vi "LoggingBlock Backup to be deleted later.vi"(8 "error in":errorcluster, 9 "Data In":T2, 11 "Queue Ref":T1) -> (0 "error out":errorcluster)   [LabVIEW 2014]
uses:
  TypeDef/Q1 Message.ctl
  <vilib>/Platform/TimedLoop/XDataNode/timing_clust.ctl
  <vilib>/Platform/TimedLoop/XDataNode/nitl_modes.ctl
  <vilib>/Platform/TimedLoop/XDataNode/wakeup.ctl
  <vilib>/platform/TimedLoop/XDataNode/XDataNode.xnode
  <vilib>/Platform/TimedLoop/XDataNode/XDNodeRunTimeDep.lvlib
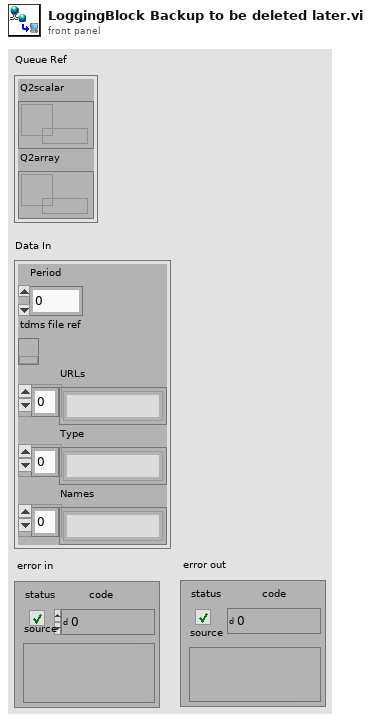
[diagram p1: front panel]
types:
  T1 = cluster{"Q2scalar":refnum<queue>, "Q2array":refnum<queue>}
  T2 = cluster{"Period":i64, "tdms file ref":refnum<k34>, "URLs":string[], "Type":string[], "Names":string[]}
  T3 = typedef "Q1 Message.ctl" = cluster{"state":enum16{"initialize 1", "initialize 2", "initialize 3", "initialize 4", "idle", "preparation", "record", "stop", "exit", "defrag", "View", "Create Database"}, "data":variant}
  T4 = typedef "XDNodeRunTimeDep.lvlib/timing_clust.ctl" = cluster{"Expected End [f-1]":u64, "Actual End [f-1]":u64, "Finished Late? [f-1]":bool, "Expected End [i-1]":u64, "Actual End [i-1]":u64, "Finished Late? [i-1]":bool, "Expected Start [i]":u64, "Actual Start [i]":u64, "Expected Start [f]":u64, "Actual Start [f]":u64, "Source Name":string, "Structure Name":string, "Period":i64, "Deadline":i64, "Offset":i64, "Start":i64, "Priority":i32, "Timeout":i32, "Mode":T5, "Wakeup Reason":T6, "Error":errorcluster, "Source Type":string, "Secondary Source Type":string, "Global End Time":u64, "Global Start Time":u64, "Frame Duration":u64, "Iteration Duration":u64, "Assigned CPU":i32, "I/O Scan Engine Mode":u32}
  T5 = typedef "XDNodeRunTimeDep.lvlib/nitl_modes.ctl" = enum32{"No Change", "Process missed periods, maintain original phase", "Discard missed periods, maintain original phase", "Process missed periods, ignore original phase", "Discard missed periods, ignore original phase"}
  T6 = typedef "XDNodeRunTimeDep.lvlib/wakeup.ctl" = enum32{"Normal", "Aborted", "Asynchronous wakeup", "Timing source error", "Timed loop error", "Timeout"}
  T7 = enum16{"initialize 1", "initialize 2", "initialize 3", "initialize 4", "idle", "preparation", "record", "stop", "exit", "defrag", "View", "Create Database"}
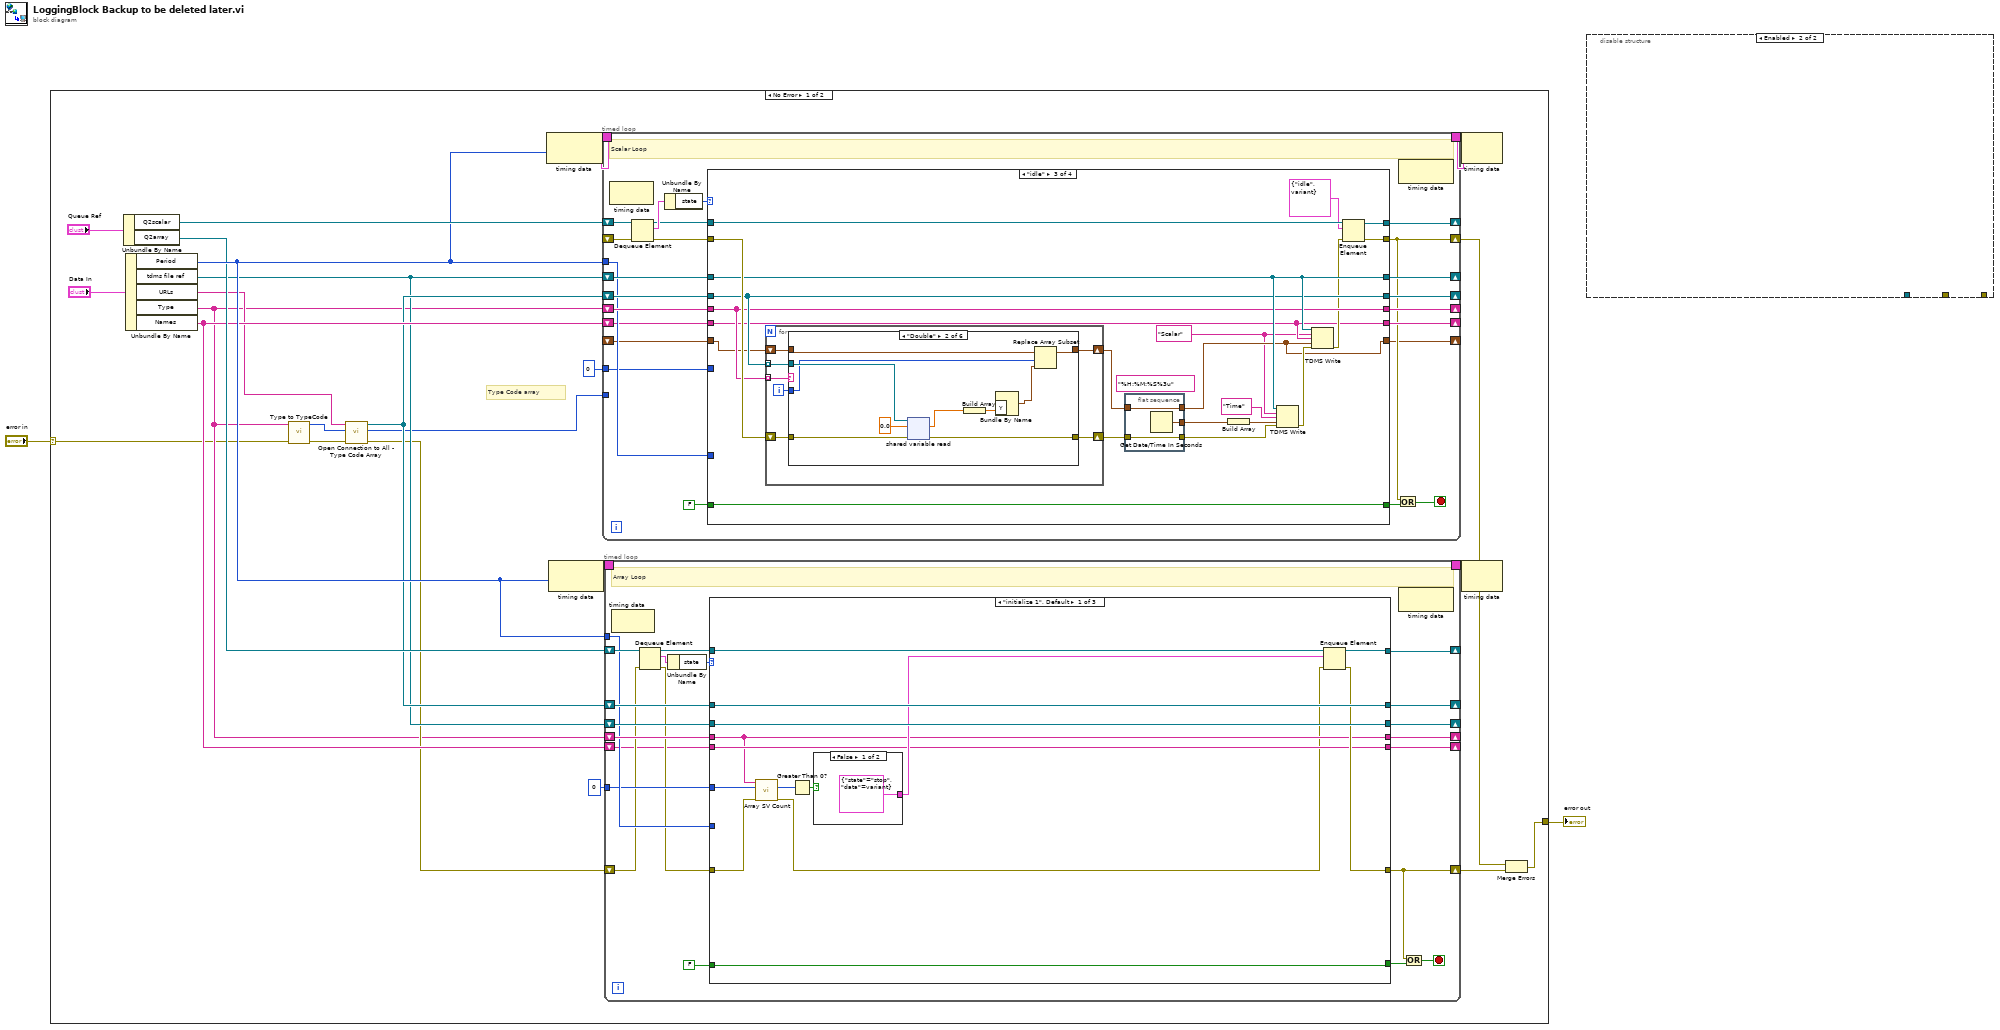
[diagram p0: block diagram]
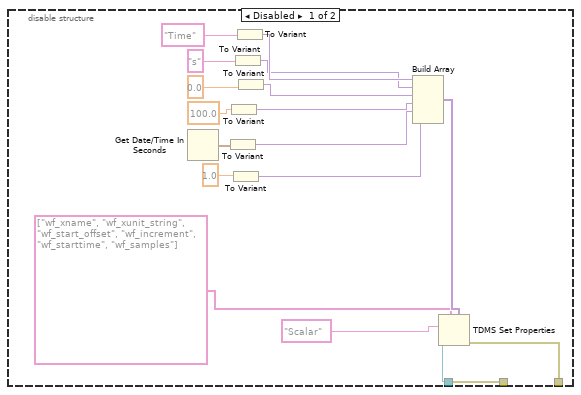
[diagram p2: hidden frame]
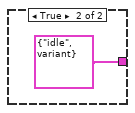
[diagram p3: hidden frame]
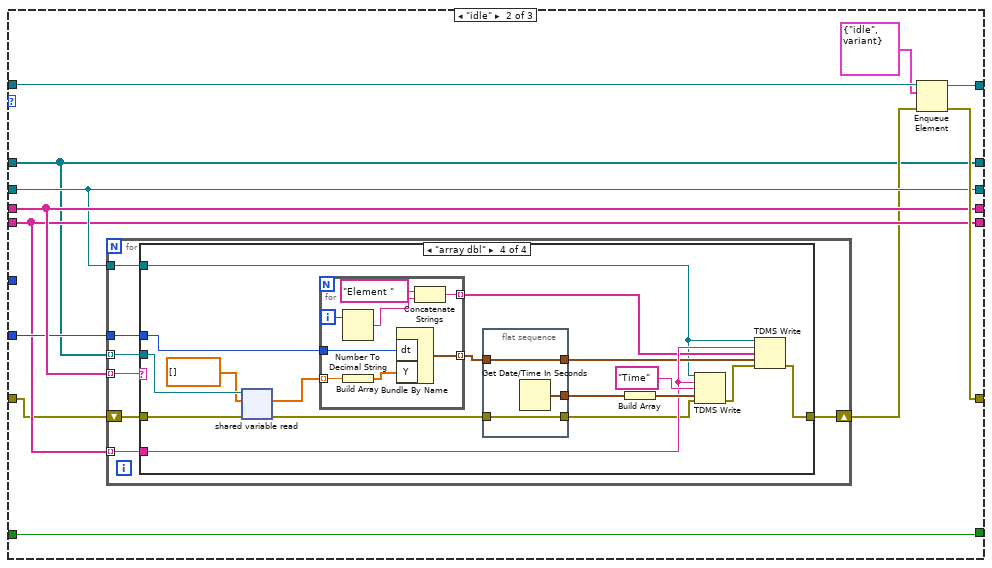
[diagram p4: hidden frame]
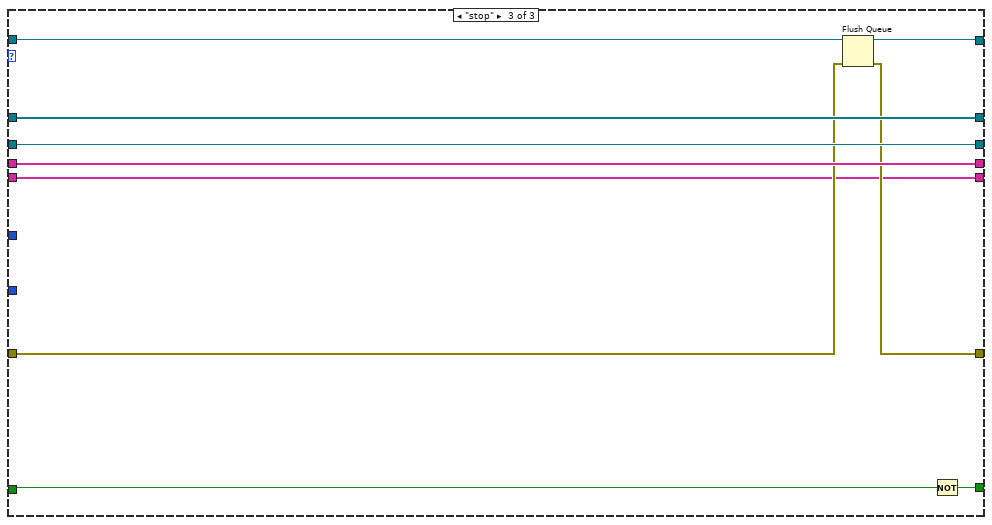
[diagram p8: hidden frame]
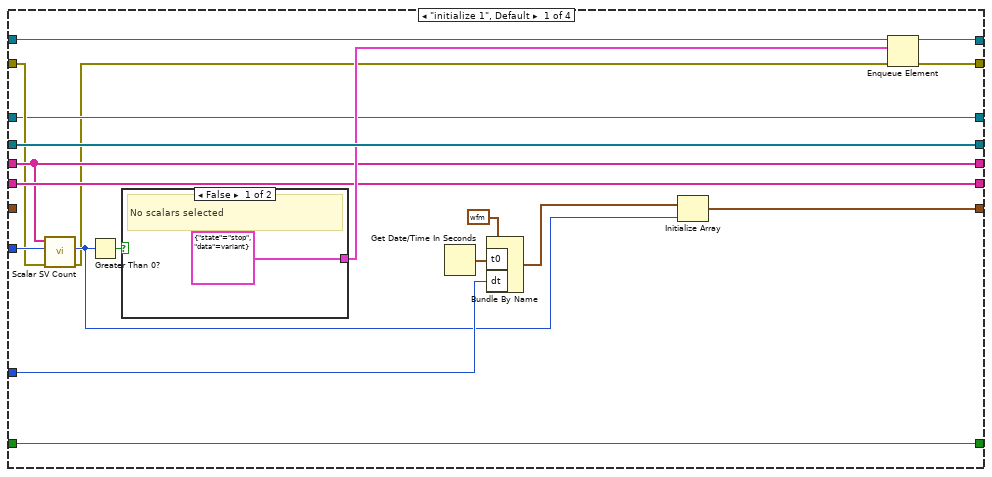
[diagram p9: hidden frame]
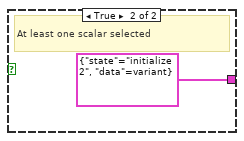
[diagram p10: hidden frame]
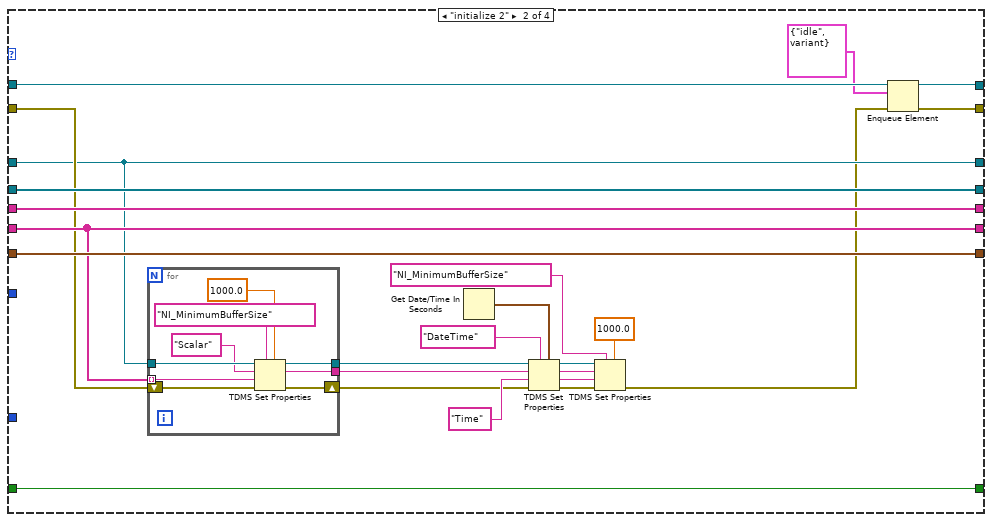
[diagram p11: hidden frame]
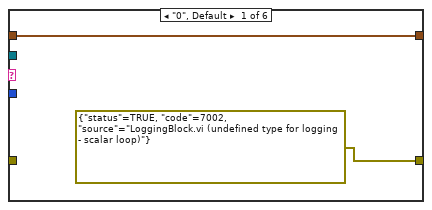
[diagram p12: hidden frame]
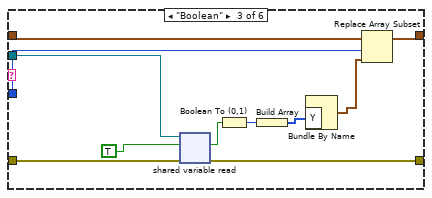
[diagram p13: hidden frame]
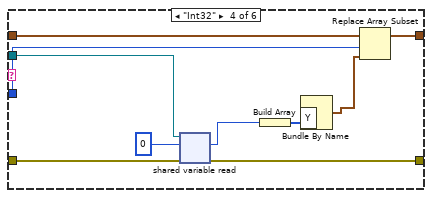
[diagram p14: hidden frame]
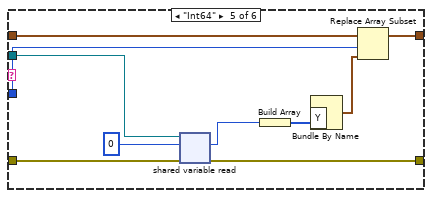
[diagram p15: hidden frame]
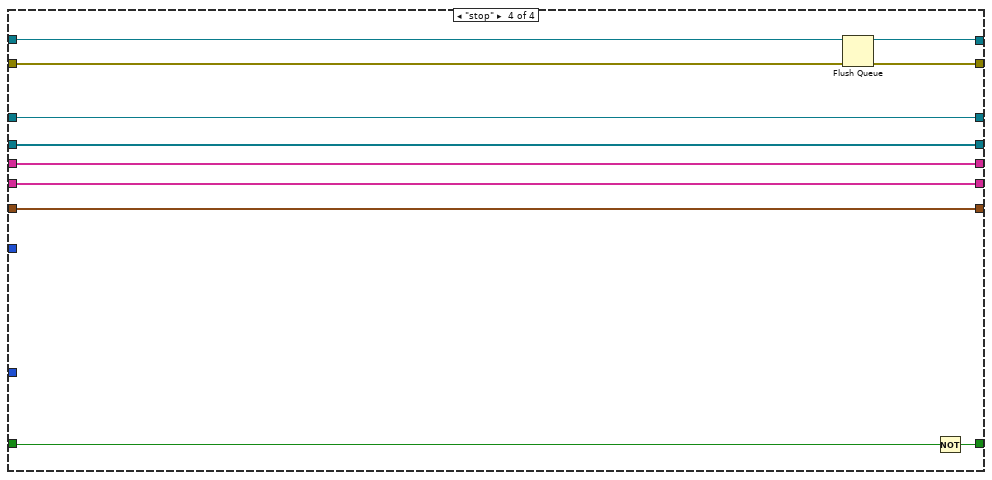
[diagram p17: hidden frame]
diagram:
  n1 = case shown="No Error" "error in" {
    selector: "error in" -> [w6 w300]
    tunnel: [w13 w300] -> w1
    frame No Error {
      # "Type Code array"
      n2 = Unbundle By Name("Queue Ref") -> ("Q2scalar"=w22:refnum<queue>, "Q2array"=w17:refnum<queue>)
      n3 = Unbundle By Name("Data In") -> ("Period"=w18:i64, "tdms file ref"=w9:refnum<k34>, "URLs"=w11:string[], "Type"=w7:string[], "Names"=w12:string[])
      n4 = call "Type to TypeCode.vi"("Error In"=w6, "Type Array"=w7) -> ("Error Out"=w5:errorcluster, "Type code Array"=w4:i32[])  [unwired: 7 in, 1 out]
      n5 = call "Open Connection to All - Type Code Array.vi"("Error In"=w5, "Type code Array"=w4, "URL array"=w11) -> ("Error Out"=w8:errorcluster, "Type code Array dup"=w3:i32[], "Array of SV Refnums"=w10:refnum<k21>[])  [unwired: 5 in, 1 out]
      n6 = node-c288(w18) -> (w24:T4)
      n7 = node-c288(w18) -> (w20:T4)
      n8 = timed-loop {
        timing: w24 -> [_]
        timing-out: [_] -> w23
        shift-right: [w143] -> _
        shift-left: w10 -> [w146]
        shift-right: [w141] -> _
        shift-left: w7 -> [w152]
        shift-right: [w144] -> _
        shift-left: w9 -> [w145]
        shift-right: [w133] -> w15
        shift-left: _ -> [w139]
        tunnel: w18 -> [w142]
        shift-right: [w147] -> _
        shift-left: w22 -> [w150]
        tunnel: 0 -> [w140]
        shift-right: [w136] -> _
        shift-left: w12 -> [w137]
        shift-right: [w131] -> _
        shift-left: _ -> [w130]
        tunnel: w3 -> [_]
        stop <- w132 stop-if-true
        # "Scalar Loop"
        n9 = node-c288() -> ()  [unwired: 1 in, 1 out]
        n10 = Dequeue Element(queue=w150, error in (no error)=w139) -> (queue out=w148:refnum<queue>, element=w151:T3, error out=w138:errorcluster)  [unwired: 1 in, 1 out]
        n11 = Unbundle By Name(w151) -> ("state"=w149:T7)
        n12 = case shown="\"idle\"" w149 {
          tunnel: w138 -> [w161 w185 w227 w289]
          tunnel: w146 -> [w169 w195 w217 w292]
          tunnel: w152 -> [w162 w192 w216 w291]
          tunnel: [w166 w194 w214 w288] -> w133
          tunnel: w148 -> [w171 w197 w221 w290]
          tunnel: [w170 w196 w220 w287] -> w147
          tunnel: [w164 w193 w210 w285] -> w134
          tunnel: [w155 w184 w218 w293] -> w144
          tunnel: w145 -> [w155 w184 w218 w293]
          tunnel: [w169 w195 w217 w292] -> w143
          tunnel: w142 -> [w157 _ _ _]
          tunnel: [w162 w192 w216 w291] -> w141
          tunnel: w140 -> [w163 _ _ _]
          tunnel: w137 -> [w165 w186 w213 w286]
          tunnel: [w165 w186 w213 w286] -> w136
          tunnel: FALSE -> [w164 w193 w210 w284]
          tunnel: [w160 w187 w208 w283] -> w131
          tunnel: w130 -> [_ w187 w209 w283]
          frame "initialize 1", Default {
            n13 = call "Scalar SV Count.vi"("Error In"=w161, "Initial number"=w163, "Type array"=w162) -> ("Error Out"=w153:errorcluster, "Number of scalar SV"=w154:i32)  [unwired: 7 in]
            n14 = Greater Than 0?(x=w154) -> (x > 0?=w168:bool)
            n15 = case shown="False" w168 {
              tunnel: [T3 {"state"=enum."stop", "data"=variant} ("Q1 Message") T3 {"state"=enum."initialize 2", "data"=variant} ("Q1 Message")] -> w167
              frame False {
                # "No scalars selected"
              }
              frame True {
                # "At least one scalar selected"
              }
            }
            n16 = Get Date/Time In Seconds() -> (seconds since 1Jan1904=w158:timestamp)
            n17 = Bundle By Name(cluster=waveform(dbl) {"t0"=timestamp(0 s since 1904-01-01), "dt"=1.0, "Y"=[]}, "t0"=w158, "dt"=w157) -> (w156:waveform(dbl))
            n18 = Initialize Array(w156, w154) -> (w160:waveform(dbl)[])
            n19 = Enqueue Element(queue=w171, element=w167, error in (no error)=w153) -> (queue out=w170:refnum<queue>, error out=w166:errorcluster)  [unwired: 1 in, 1 out]
          }
          frame "initialize 2" {
            n20 = for {
              tunnel: w186 -> [w206] mode=indexing
              tunnel: w184 -> [w204]
              shift-right: [w200] -> w182
              shift-left: w185 -> [w205]
              tunnel: [w199] -> w183
              tunnel: [w198] -> w180
              n21 = TDMS Set Properties(5:1000.0, 7:"NI_MinimumBufferSize", 8:w205, 9:w206, 10:"Scalar", 11:w204) -> (0:w200:errorcluster, 2:w199:string, 3:w198:refnum<k34>)  [unwired: 1 out]
            }
            n22 = Get Date/Time In Seconds() -> (seconds since 1Jan1904=w190:timestamp)
            n23 = TDMS Set Properties(5:w190, 7:"DateTime" ("property names"), 8:w182, 9:"Time", 10:w183, 11:w180) -> (0:w177:errorcluster, 1:w178:string, 2:w179:string, 3:w181:refnum<k34>)
            n24 = TDMS Set Properties(5:1000.0, 7:"NI_MinimumBufferSize", 8:w177, 9:w178, 10:w179, 11:w181) -> (0:w174:errorcluster)  [unwired: 3 out]
            n25 = Enqueue Element(queue=w197, element=T3 {"state"=enum."idle", "data"=variant} ("Q1 Message"), error in (no error)=w174) -> (queue out=w196:refnum<queue>, error out=w194:errorcluster)  [unwired: 1 in, 1 out]
          }
          frame "idle" {
            (unwired) "%H:%M:%S%3u" ("time format string (%c)")
            w207 = "Scalar"
            n26 = for {
              tunnel: w217 -> [w237] mode=indexing
              tunnel: w216 -> [w232] mode=indexing
              shift-right: [w235] -> w226
              shift-left: w227 -> [w236]
              shift-right: [w233] -> w225
              shift-left: w209 -> [w234]
              i -> [w231]
              n27 = case shown="\"Double\"" w232 {
                tunnel: w237 -> [_ w244 w258 w263 w275 _]
                tunnel: w236 -> [_ w246 w260 w267 w277 w281]
                tunnel: [errorcluster {"status"=TRUE, "code"=7002, "source"="LoggingBlock.vi (undefined type for logging - scalar loop)"} ("error out") w245 w259 w266 w276 w281] -> w235
                tunnel: w234 -> [w239 w242 w256 w264 w272 w282]
                tunnel: [w239 w243 w257 w265 w271 w282] -> w233
                tunnel: w231 -> [_ w241 w255 w261 w273 _]
                frame "0", Default {
                }
                frame "Double" {
                  n28 = shared-variable-read(w244, w246, 0.0) -> (w245:errorcluster, w247:dbl)  [unwired: 2 out]
                  n29 = Build Array(w247) -> (w248:dbl[])
                  n30 = Bundle By Name("Y"=w248) -> (w240:waveform(dbl))  [unwired: 1 in]
                  n31 = Replace Array Subset(array=w242, new element=w240, index=w241) -> (w243:waveform(dbl)[])
                }
                frame "Boolean" {
                  n32 = shared-variable-read(w258, w260, TRUE) -> (w259:errorcluster, w251:bool)  [unwired: 2 out]
                  n33 = Boolean To (0,1)(Boolean=w251) -> (0, 1=w252:i16)
                  n34 = Build Array(w252) -> (w250:i16[])
                  n35 = Bundle By Name("Y"=w250) -> (w254:waveform(i16))  [unwired: 1 in]
                  n36 = Replace Array Subset(array=w256, new element=w254, index=w255) -> (w257:waveform(dbl)[])
                }
                frame "Int32" {
                  n37 = shared-variable-read(w263, w267, 0) -> (w266:errorcluster, w268:i32)  [unwired: 2 out]
                  n38 = Build Array(w268) -> (w269:i32[])
                  n39 = Bundle By Name("Y"=w269) -> (w262:waveform(i32))  [unwired: 1 in]
                  n40 = Replace Array Subset(array=w264, new element=w262, index=w261) -> (w265:waveform(dbl)[])
                }
                frame "Int64" {
                  n41 = shared-variable-read(w275, w277, i64 0) -> (w276:errorcluster, w278:i64)  [unwired: 2 out]
                  n42 = Build Array(w278) -> (w279:i64[])
                  n43 = Bundle By Name("Y"=w279) -> (w274:waveform(i64))  [unwired: 1 in]
                  n44 = Replace Array Subset(array=w272, new element=w274, index=w273) -> (w271:waveform(dbl)[])
                }
                frame "1D array of Double" {
                }
              }
            }
            n45 = flat-sequence {
              tunnel: w226 -> [w229]
              tunnel: w225 -> [w228]
              tunnel: [w230] -> w212
              tunnel: [w229] -> w223
              tunnel: [w228] -> w208
              frame #0 {
                n46 = Get Date/Time In Seconds() -> (seconds since 1Jan1904=w230:timestamp)
              }
            }
            n47 = Build Array(w212) -> (w211:timestamp[])
            n48 = TDMS Write(0:w218, 5:w207, 7:"Time", 9:w211, 11:w223) -> (15:w222:errorcluster)  [unwired: 1 in, 3 out]
            n49 = TDMS Write(0:w218, 5:w207, 7:w213, 9:w208, 11:w222) -> (15:w215:errorcluster)  [unwired: 1 in, 3 out]
            n50 = Enqueue Element(queue=w221, element=T3 {"state"=enum."idle", "data"=variant} ("Q1 Message"), error in (no error)=w215) -> (queue out=w220:refnum<queue>, error out=w214:errorcluster)  [unwired: 1 in, 1 out]
          }
          frame "stop" {
            n51 = Flush Queue(queue=w290, error in (no error)=w289) -> (queue out=w287:refnum<queue>, error out=w288:errorcluster)  [unwired: 1 out]
            n52 = Not(x=w284) -> (.not. x?=w285:bool)
          }
        }
        n53 = Or(x=w133, y=w134) -> (x .or. y?=w132:bool)
        n54 = node-c288() -> ()  [unwired: 1 in, 1 out]
      }
      n55 = timed-loop {
        timing: w20 -> [_]
        timing-out: [_] -> w19
        shift-right: [w38] -> _
        shift-left: w9 -> [w41]
        shift-right: [w36] -> _
        shift-left: w7 -> [w47]
        shift-right: [w39] -> _
        shift-left: w10 -> [w40]
        shift-right: [w28] -> w14
        shift-left: w8 -> [w33]
        tunnel: w18 -> [w37]
        shift-right: [w42] -> _
        shift-left: w17 -> [w45]
        tunnel: 0 -> [w35]
        shift-right: [w31] -> _
        shift-left: w12 -> [w32]
        stop <- w27 stop-if-true
        # "Array Loop"
        n56 = node-c288() -> ()  [unwired: 1 in, 1 out]
        n57 = Dequeue Element(queue=w45, error in (no error)=w33) -> (queue out=w43:refnum<queue>, element=w46:T3, error out=w34:errorcluster)  [unwired: 1 in, 1 out]
        n58 = Unbundle By Name(w46) -> ("state"=w44:T7)
        n59 = case shown="\"initialize 1\", Default" w44 {
          tunnel: w34 -> [w50 w67 w119]
          tunnel: w41 -> [w58 w69 w122]
          tunnel: w47 -> [w52 w71 w121]
          tunnel: [w55 w72 w118] -> w28
          tunnel: w43 -> [w61 w75 w120]
          tunnel: [w60 w74 w117] -> w42
          tunnel: [w59 w65 w123] -> w39
          tunnel: w40 -> [w59 w65 w123]
          tunnel: [w58 w69 w122] -> w38
          tunnel: w37 -> [_ w70 _]
          tunnel: [w52 w71 w121] -> w36
          tunnel: w35 -> [w51 _ _]
          tunnel: w32 -> [w54 w68 w116]
          tunnel: [w54 w68 w116] -> w31
          tunnel: FALSE -> [w53 w64 w115]
          tunnel: [w53 w64 w114] -> w29
          frame "initialize 1", Default {
            n60 = call "Array SV Count.vi"("Error In"=w50, "Initial number"=w51, "Type array"=w52) -> ("Error Out"=w49:errorcluster, "Number of scalar SV"=w48:i32)  [unwired: 7 in]
            n61 = Greater Than 0?(x=w48) -> (x > 0?=w57:bool)
            n62 = case shown="False" w57 {
              tunnel: [T3 {"state"=enum."stop", "data"=variant} ("Q1 Message") T3 {"state"=enum."idle", "data"=variant} ("Q1 Message")] -> w56
              frame False {
              }
              frame True {
              }
            }
            n63 = Enqueue Element(queue=w61, element=w56, error in (no error)=w49) -> (queue out=w60:refnum<queue>, error out=w55:errorcluster)  [unwired: 1 in, 1 out]
          }
          frame "idle" {
            n64 = for {
              tunnel: w65 -> [w81] mode=indexing
              tunnel: w71 -> [w82] mode=indexing
              shift-right: [w79] -> w66
              shift-left: w67 -> [w80]
              tunnel: w70 -> [w78]
              tunnel: w68 -> [w77] mode=indexing
              tunnel: w69 -> [w76]
              n65 = case shown="\"array dbl\"" w82 {
                tunnel: w81 -> [_ _ _ w101]
                tunnel: w80 -> [w83 w84 w85 w100]
                tunnel: [w83 w84 w85 w89] -> w79
                tunnel: w78 -> [_ _ _ w99]
                tunnel: w77 -> [_ _ _ w93]
                tunnel: w76 -> [_ _ _ w88]
                frame "dbl", Default {
                }
                frame "int32" {
                }
                frame "int64" {
                }
                frame "array dbl" {
                  n66 = shared-variable-read(w101, w100, dbl[] []) -> (w97:errorcluster, w102:dbl[])  [unwired: 2 out]
                  n67 = for {
                    tunnel: w102 -> [w113] mode=indexing
                    tunnel: w99 -> [w112]
                    tunnel: [w111] -> w96 mode=indexing
                    tunnel: [w106] -> w92 mode=indexing
                    i -> [w109]
                    n68 = Number To Decimal String(number=w109) -> (decimal integer string=w107:string)  [unwired: 1 in]
                    n69 = Build Array(w113) -> (w110:dbl[])
                    n70 = Bundle By Name("dt"=w112, "Y"=w110) -> (w111:waveform(dbl))  [unwired: 1 in]
                    n71 = Concatenate Strings("Element ", w107) -> (w106:string)
                  }
                  n72 = flat-sequence {
                    tunnel: w97 -> [w105]
                    tunnel: w96 -> [w104]
                    tunnel: [w105] -> w87
                    tunnel: [w104] -> w90
                    tunnel: [w103] -> w86
                    frame #0 {
                      n73 = Get Date/Time In Seconds() -> (seconds since 1Jan1904=w103:timestamp)
                    }
                  }
                  n74 = Build Array(w86) -> (w95:timestamp[])
                  n75 = TDMS Write(0:w88, 5:w93, 7:"Time", 9:w95, 11:w87) -> (15:w91:errorcluster)  [unwired: 1 in, 3 out]
                  n76 = TDMS Write(0:w88, 5:w93, 7:w92, 9:w90, 11:w91) -> (15:w89:errorcluster)  [unwired: 1 in, 3 out]
                }
              }
            }
            n77 = Enqueue Element(queue=w75, element=T3 {"state"=enum."idle", "data"=variant} ("Q1 Message"), error in (no error)=w66) -> (queue out=w74:refnum<queue>, error out=w72:errorcluster)  [unwired: 1 in, 1 out]
          }
          frame "stop" {
            n78 = Flush Queue(queue=w120, error in (no error)=w119) -> (queue out=w117:refnum<queue>, error out=w118:errorcluster)  [unwired: 1 out]
            n79 = Not(x=w115) -> (.not. x?=w114:bool)
          }
        }
        n80 = node-c288() -> ()  [unwired: 1 in, 1 out]
        n81 = Or(x=w28, y=w29) -> (x .or. y?=w27:bool)
      }
      n82 = node-c288(w23) -> ()  [unwired: 1 out]
      n83 = node-c288(w19) -> ()  [unwired: 1 out]
      n84 = Merge Errors(w15, w14) -> (w13:errorcluster)
    }
    frame Error {
    }
  }
  "error out" <- w1
  n85 = disable-structure shown="Enabled" {
    disable-tunnel: _ -> [w304 _]
    disable-tunnel: [w302 _] -> _
    disable-tunnel: _ -> [w301 _]
    frame Disabled {
      n86 = Get Date/Time In Seconds() -> (seconds since 1Jan1904=w316:timestamp)
      n87 = To Variant(anything=w316) -> (Variant=w308:variant)
      n88 = To Variant(anything=100.0) -> (Variant=w309:variant)
      n89 = To Variant(anything=1.0) -> (Variant=w307:variant)
      n90 = To Variant(anything="s" ("name")) -> (Variant=w311:variant)
      n91 = To Variant(anything="Time" ("name")) -> (Variant=w312:variant)
      n92 = To Variant(anything=0.0) -> (Variant=w310:variant)
      n93 = Build Array(w312, w311, w310, w309, w308, w307) -> (w306:variant[])
      n94 = TDMS Set Properties(5:w306, 7:string[] ["wf_xname", "wf_xunit_string", "wf_start_offset", "wf_increment", "wf_starttime", "wf_samples"], 8:w301, 10:"Scalar", 11:w304) -> (0:w302:errorcluster)  [unwired: 1 in, 3 out]
    }
    frame Enabled {
    }
  }
